vi "SW_Generate_Segmented_Plot_v3b.vi"() -> ()   [LabVIEW 2016]
panel:
  out "Pixels per mm":dbl
  out "Radius of displayed outer segments, pix":dbl
  out "Zones display background":picture
  in  "Scale factor for outer display radius display":dbl=0.95 format="%#_13g"
  out "Fonts scale factor":dbl
  in  "Input cluster of parameters":T1={"Amount of border segments"=8, "Border segments starting angle"=0, "Amount of midfield segments"=4, "Midfield segments starting angle"=0, "Midfield segments outer radius, mm"=60, "Amount of central segments"=1, "Center segment outer radius, mm"=30, "Diameter of the cage, mm"=180, "R-gap between segments, mm"=10} {"Diameter of the cage, mm" scale=20.0..250.0}
  in  "Fill color for no segments image":u32(colorbox)=6316128
  out "Error Out":errorcluster
  in  "Error In":errorcluster
  in  "Color for central segment":u32=16777113
  in  "Colors array for midfield segments":u32[](array[numeric])=[8073876, 10935200, 34871, 12756431]
  in  "Colors array for outer segments":u32[](array[numeric])=[14102567, 16625249, 14742520, 7646673, 16018755, 16703632, 11262441, 4552116]
  in  "Background color":u32(colorbox)=13816530
  in  "Draw Area Size":cluster{"Width":dbl, "Height":dbl}={"Width"=480.0, "Height"=480.0}
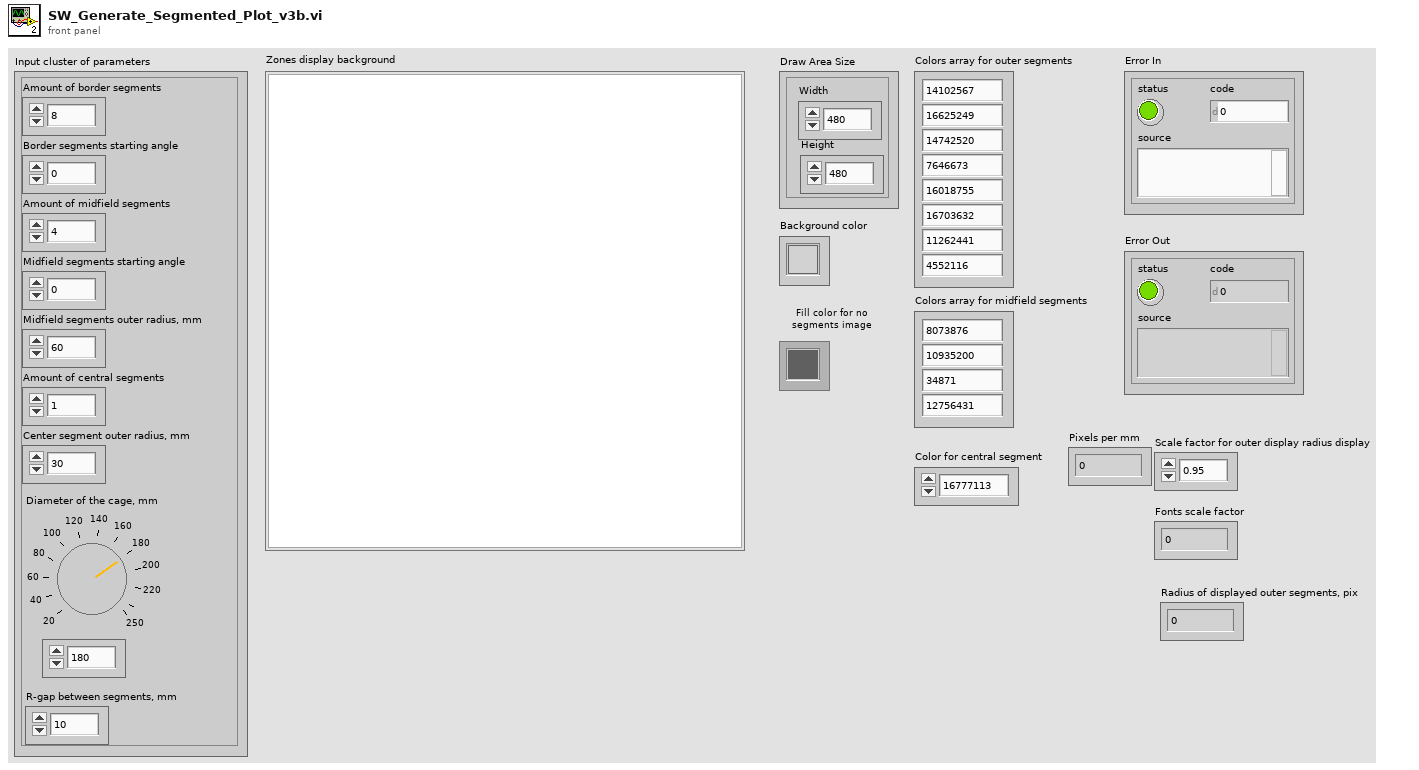
[diagram p1: front panel]
types:
  T1 = cluster{"Amount of border segments":u8, "Border segments starting angle":i16, "Amount of midfield segments":u8, "Midfield segments starting angle":i16, "Midfield segments outer radius, mm":u16, "Amount of central segments":u8, "Center segment outer radius, mm":u16, "Diameter of the cage, mm":u16, "R-gap between segments, mm":u8}
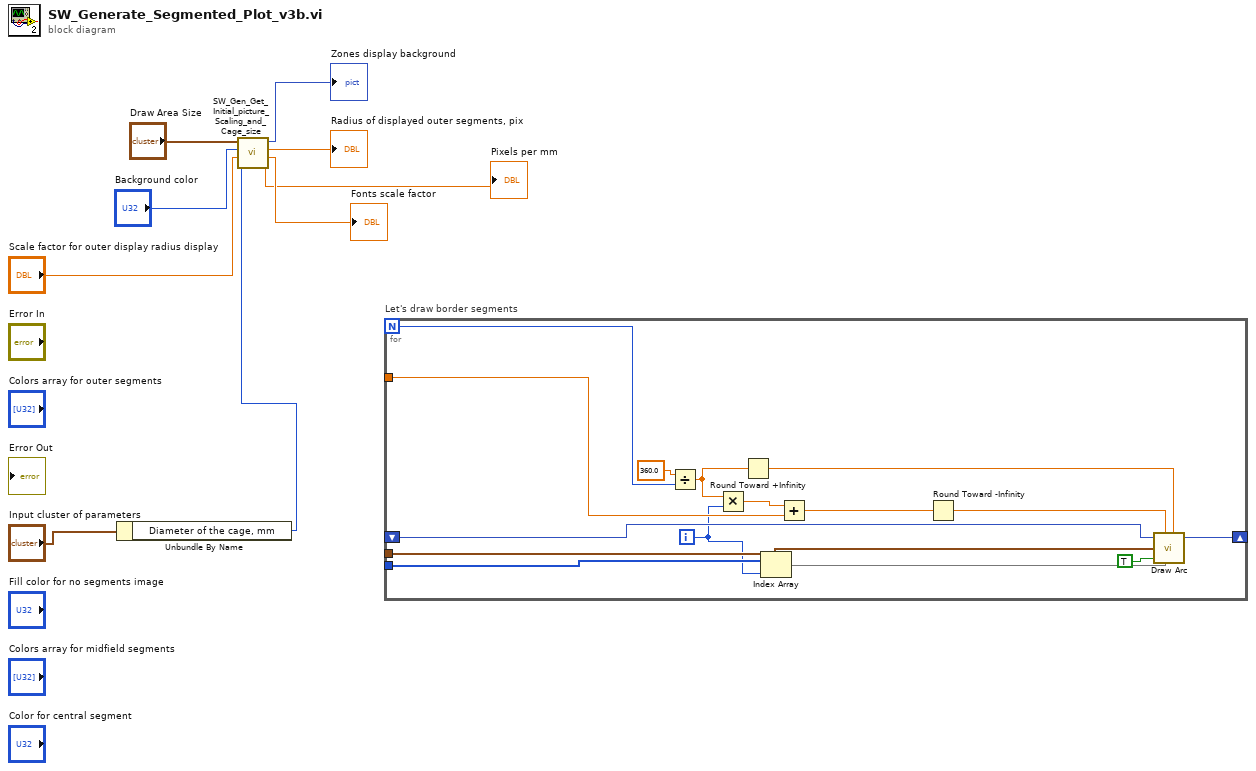
[diagram p0: block diagram]
diagram:
  n1 = Unbundle By Name("Input cluster of parameters") -> ("Diameter of the cage, mm"=w2:u16)
  n2 = call "SW_Gen_Get_Initial_picture_Scaling_and_Cage_size.vi"("Diameter of the cage, mm"=w2, "Scale factor for outer display radius display"="Scale factor for outer display radius display", "Background color"="Background color", "Draw Area Size"="Draw Area Size") -> ("Pixels per mm"=→"Pixels per mm":dbl, "Fonts scale factor"=→"Fonts scale factor":dbl, "Radius of displayed outer segments, pix"=→"Radius of displayed outer segments, pix":dbl, "Zones display background"=→"Zones display background":picture)  [unwired: 4 in]
  n3 = for "Let's draw border segments" {
    N -> [w16]
    tunnel: _ -> [w21]
    shift-right: [w14] -> _
    shift-left: _ -> [w23]
    tunnel: _ -> [w17]
    tunnel: _ -> [w20]
    i -> [w11]
    n4 = Divide(x=360.0, y=w16) -> (x/y=w15:dbl)
    n5 = Multiply(x=w15, y=w11) -> (x*y=w22:dbl)
    n6 = Round Toward +Infinity(x=w15) -> (ceil(x): smallest int >= x=w13:dbl)
    n7 = Index Array(array=w20, index=w11) -> (element=w10)
    n8 = Add(x=w22, y=w21) -> (x+y=w18:dbl)
    n9 = Round Toward -Infinity(1:w18) -> (0:w12:dbl)
    n10 = call <vilib>:"Draw Arc.vi"("picture"=w23, "start angle[degrees]"=w12, "rect"=w17, "fill?(F)"=TRUE, "color(black)"=w10, "arc size[degrees]"=w13) -> ("new picture"=w14:picture)  [unwired: 3 in]
  }
